vi "To Serial Form.vi"(6 "Serial Version":T1, 10 "Serializer in":refnum<class "Serializer.lvclass">, 11 "Alicat Controller in":refnum<class "Alicat Controller.lvclass">) -> (0 "error out":errorcluster, 2 "Serializer out":refnum<class "Serializer.lvclass">, 3 "Alicat Controller out":refnum<class "Alicat Controller.lvclass">)   [LabVIEW 2012, in "Alicat.lvlib" / "Alicat Controller.lvclass"]
uses:
  Alicat Controller.lvclass
  <userlib>/Serialization/Serializer/Serializer.lvclass
  <userlib>/Serialization/Serialization Common/Serial Version.ctl
  Alicat.lvclass
  Alicat Controller.lvclass/Alicat Controller.ctl
  <userlib>/Serialization/Serializer/Serializer.lvclass/Serializer.ctl
  <userlib>/Serialization/Formatter/Formatter.lvclass/Formatter.ctl
  <userlib>/Serialization/Serializable/Insert Single.vi
  <userlib>/Serialization/Serializer/Insert Single.vi
  <userlib>/Serialization/Formatter/Read Include all fields.vi
  <userlib>/Serialization/Serializable/Serializable.lvclass
  <userlib>/Serialization/Serialization Common/Serialization Common.lvlib
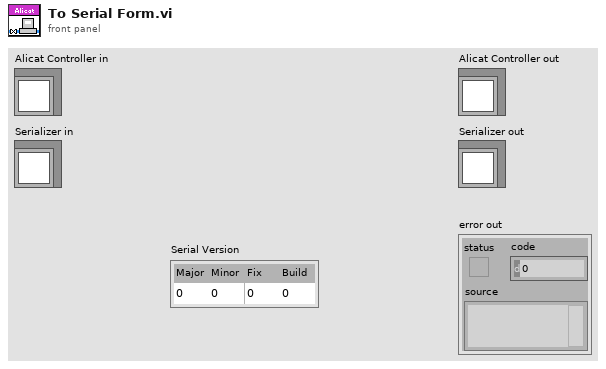
[diagram p1: front panel]
types:
  T1 = typedef "Serialization Common.lvlib/Serial Version.ctl" = cluster{"Major":u16, "Minor":u16, "Fix":u16, "Build":u16}
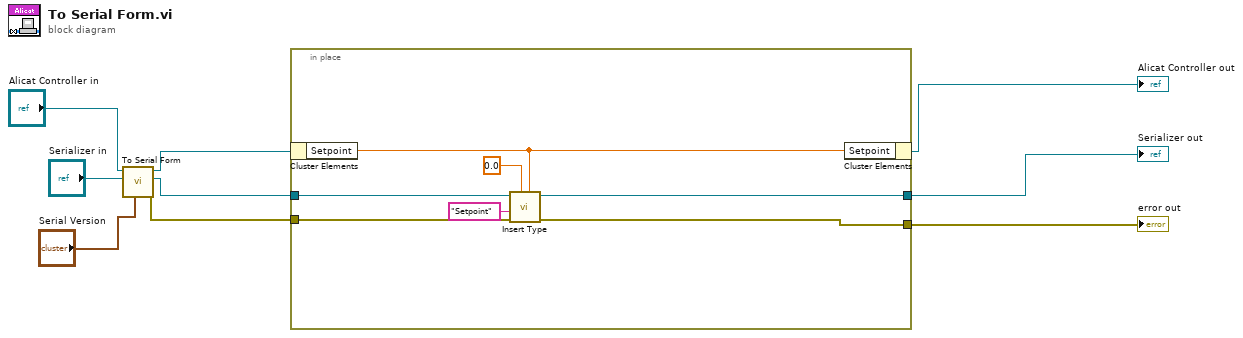
[diagram p0: block diagram]
diagram:
  n1 = call-parent "To Serial Form.vi"("Serial Version"="Serial Version", "Serializer in"="Serializer in", "Alicat in"="Alicat Controller in") -> ("error out"=w4:errorcluster, "Serializer out"=w5:refnum<class "Serializer.lvclass">, "Alicat out"=w6:refnum<class "Alicat Controller.lvclass">)  [unwired: 6 in]
  n2 = in-place {
    in-place-border: w5 -> [w15]
    in-place-border: w4 -> [w14]
    in-place-border: [w13] -> w3
    in-place-border: [w12] -> w1
    n3 = in-place-cluster #1(w6) -> ("Setpoint"=w11:sgl)
    n4 = call-poly <userlib>:"Insert Type.vi"("Double"=w11, "Default Value"=sgl 0.0, "error in (no error)"=w14, "Name"="Setpoint", "Serializer in"=w15) -> ("error out"=w12:errorcluster, "Serializer out"=w13:refnum<class "Serializer.lvclass">)  [unwired: 5 in]
    n5 = in-place-cluster #1("Setpoint"=w11) -> (→"Alicat Controller out":refnum<class "Alicat Controller.lvclass">)
  }
  "error out" <- w1
  "Serializer out" <- w3
